vi "DC Transport Configure.vi"(0 "Channel 2":bool, 3 "Channel 1":bool=TRUE, 4 "Voltmeter Buffer Size":string="62", 5 "Voltmeter 2 Address":string="8", 6 "Voltmeter Range (V)":string="0.01", 7 "Voltmeter 1 Address":string="7", 8 "NPLC":string="1", 9 "Time Period (s)":string="3", 10 "Current Amplitude":string="1e-10", 11 "6221 Address":string="12") -> ()   [LabVIEW 2020]
panel:
  out "2182A Input Command":string="*RST\n:SYSTem:AZERo:STATe OFF\n:SENSe:VOLTage:DC:LPASs OFF\n:SENSe:VOLTage:DC:DFILter OFF\n:SENSe:VOLTage:DC:RANGe 0.01\n:form:elem read, tst\n:disp:enab ON\n:sens:volt:nplc 1\n:trig:sour imm\n:init:cont off\n:abort\n:trac:clear\n:trac:poin 62\n:trac:feed sens\n:trac:feed:cont next"
  in  "INIT Wave":bool
  out "6221 Commands":string="*RST\nSOUR:WAVE:ARB:DATA 1,-1\nSOUR:WAVE:ARB:COPY 4\nSOUR:WAVE:FUNC ARB4\nSOUR:WAVE:AMPL 1e-10\nSOUR:WAVE:FREQ 3.333333E-1\nSOUR:WAVE:OFFS 0\nOUTPUT:LTEARTH ON\nSOUR:WAVE:PMAR:STAT OFF\nSOUR:WAVE:RANG BEST\nSOUR:CURR:COMP 1\nSOUR:WAVE:DUR:TIME 3\nSOUR:WAVE:ARM"
  in  "INF Wave":bool
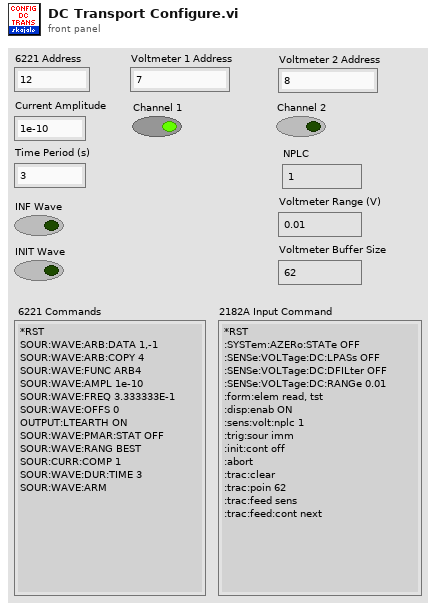
[diagram p1: front panel]
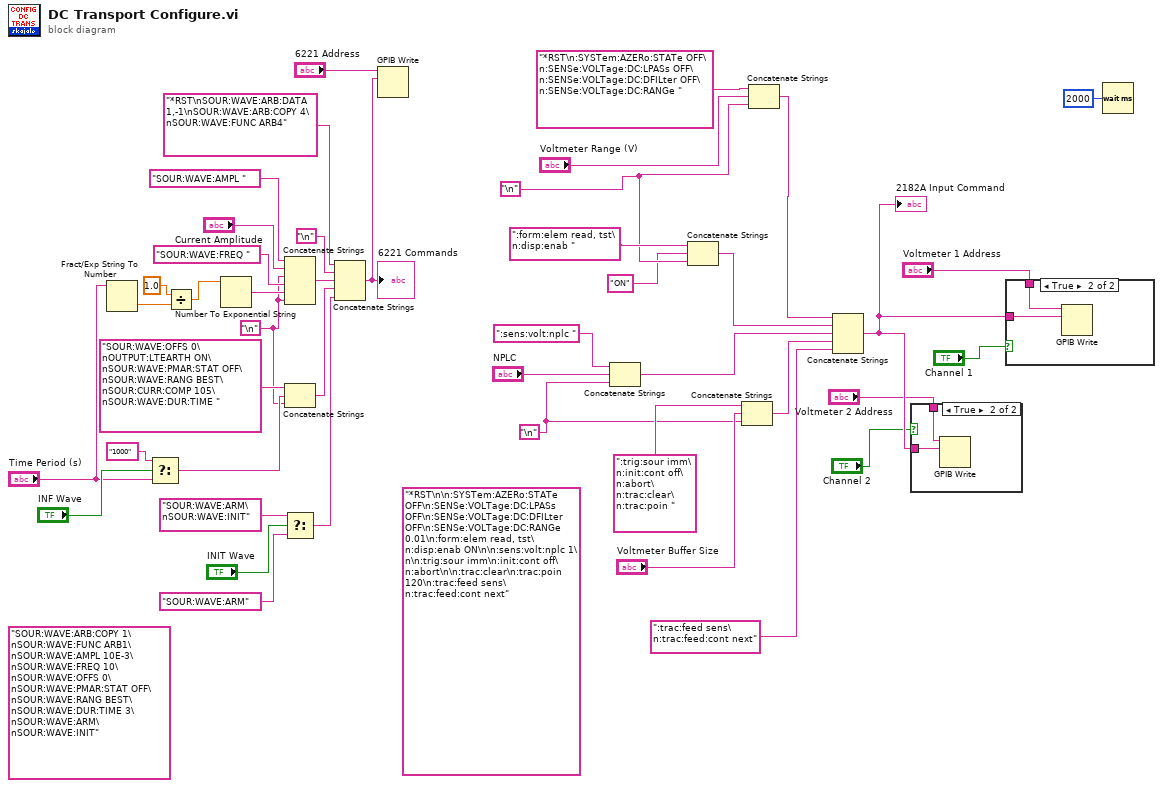
[diagram p0: block diagram]
diagram:
  w8 = "\n"
  (unwired) "*RST\n\n:SYSTem:AZERo:STATe OFF\n:SENSe:VOLTage:DC:LPASs OFF\n:SENSe:VOLTage:DC:DFILter OFF\n:SENSe:VOLTage:DC:RANGe 0.01\n:form:elem read, tst\n:disp:enab ON\n\n:sens:volt:nplc 1\n\n:trig:sour imm\n:init:cont off\n:abort\n\n:trac:clear\n:trac:poin 120\n:trac:feed sens\n:trac:feed:cont next"
  w10 = "\n"
  w24 = "\n"
  (unwired) "SOUR:WAVE:ARB:COPY 1\nSOUR:WAVE:FUNC ARB1\nSOUR:WAVE:AMPL 10E-3\nSOUR:WAVE:FREQ 10\nSOUR:WAVE:OFFS 0\nSOUR:WAVE:PMAR:STAT OFF\nSOUR:WAVE:RANG BEST\nSOUR:WAVE:DUR:TIME 3\nSOUR:WAVE:ARM\nSOUR:WAVE:INIT" ("data")
  n1 = Fract/Exp String To Number(string="Time Period (s)") -> (number=w29:dbl)  [unwired: 3 in, 1 out]
  n2 = Select(t="1000", s="INF Wave", f="Time Period (s)") -> (s? t:f=w36:string)
  n3 = Divide(x=1.0, y=w29) -> (x/y=w40:dbl)
  n4 = Number To Exponential String(number=w40) -> (E-format string=w39:string)  [unwired: 3 in]
  n5 = Concatenate Strings("SOUR:WAVE:AMPL ", "Current Amplitude", w24, "SOUR:WAVE:FREQ ", w39, w24) -> (w33:string)
  n6 = Concatenate Strings("SOUR:WAVE:OFFS 0\nOUTPUT:LTEARTH ON\nSOUR:WAVE:PMAR:STAT OFF\nSOUR:WAVE:RANG BEST\nSOUR:CURR:COMP 105\nSOUR:WAVE:DUR:TIME ", w36, w24) -> (w32:string)
  n7 = Select(t="SOUR:WAVE:ARM\nSOUR:WAVE:INIT" ("string"), s="INIT Wave", f="SOUR:WAVE:ARM" ("string")) -> (s? t:f=w27:string)
  n8 = Concatenate Strings("*RST\nSOUR:WAVE:ARB:DATA 1,-1\nSOUR:WAVE:ARB:COPY 4\nSOUR:WAVE:FUNC ARB4", "\n", w33, w32, w27) -> (w31:string)
  "6221 Commands" <- w31
  n9 = GPIB Write(0:"6221 Address", 1:w31) -> ()  [unwired: 3 in, 2 out]
  n10 = Concatenate Strings(":sens:volt:nplc ", "NPLC", w8) -> (w13:string)
  n11 = Concatenate Strings(":form:elem read, tst\n:disp:enab ", "ON" ("string"), w10) -> (w14:string)
  n12 = Concatenate Strings(":trig:sour imm\n:init:cont off\n:abort\n:trac:clear\n:trac:poin ", "Voltmeter Buffer Size", w8) -> (w12:string)
  n13 = Concatenate Strings("*RST\n:SYSTem:AZERo:STATe OFF\n:SENSe:VOLTage:DC:LPASs OFF\n:SENSe:VOLTage:DC:DFILter OFF\n:SENSe:VOLTage:DC:RANGe ", "Voltmeter Range (V)", w10) -> (w15:string)
  n14 = Concatenate Strings(w15, w14, w13, w12, ":trac:feed sens\n:trac:feed:cont next") -> (w6:string)
  "2182A Input Command" <- w6
  n15 = case shown="True" "Channel 2" {
    tunnel: w6 -> [_ w46]
    tunnel: "Voltmeter 2 Address" -> [_ w45]
    frame False {
    }
    frame True {
      n16 = GPIB Write(0:w45, 1:w46) -> ()  [unwired: 3 in, 2 out]
    }
  }
  n17 = case shown="True" "Channel 1" {
    tunnel: "Voltmeter 1 Address" -> [_ w48]
    tunnel: w6 -> [_ w47]
    frame False {
    }
    frame True {
      n18 = GPIB Write(0:w48, 1:w47) -> ()  [unwired: 3 in, 2 out]
    }
  }
  n19 = Wait (ms)(milliseconds to wait=u32 2000) -> ()  [unwired: 1 out]
